vi "Analyze.vi"(8 "error in (no error)":errorcluster, 10 "Image in":T1, 11 "Analyze SecondMomentum in":refnum<class "Analyze SecondMomentum.lvclass">) -> (0 "error out":errorcluster, 1 "Result":refnum<class "Analyze Results Base.lvclass">, 2 "Image out":T1, 3 "Analyze SecondMomentum out":refnum<class "Analyze SecondMomentum.lvclass">)   [LabVIEW 2014, in "Analyze.lvlib" / "Analyze SecondMomentum.lvclass"]
uses:
  Analyze SecondMomentum.lvclass
  <vilib>/vision/Image Controls.llb/IMAQ Image.ctl
  Results and Overlays/Results Base/Analyze Results Base.lvclass
  Results and Overlays/Results Second Momentum/Analyze Results Second Momentum.lvclass
  Results and Overlays/Results Second Momentum/Analyze Results Second Momentum.lvclass/Analyze Results Second Momentum.ctl
  Results and Overlays/Results Second Momentum/Write 1st M x 1.vi
  Results and Overlays/Results Second Momentum/Write 1st M y 1.vi
  Results and Overlays/Results Second Momentum/Write 2nd M x 1.vi
  Results and Overlays/Results Second Momentum/Write 2nd M y 1.vi
  Results and Overlays/Results Second Momentum/Write D x 1.vi
  Analyze BaseClass/Analyze BaseClass/Analyze BaseClass.lvclass
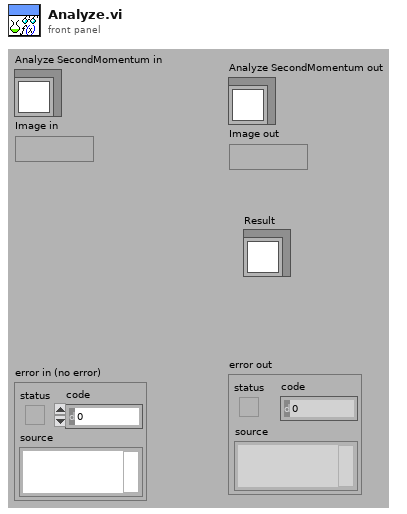
[diagram p1: front panel]
types:
  T1 = typedef "IMAQ Image.ctl" = refnum<image>
  T2 = typedef "ROI Descriptor" = cluster{"Global Rectangle":i32[], "Contours":cluster{"ID":enum32{"External", "Internal"}, "Type":u32, "Coordinates":i32[]}[]}
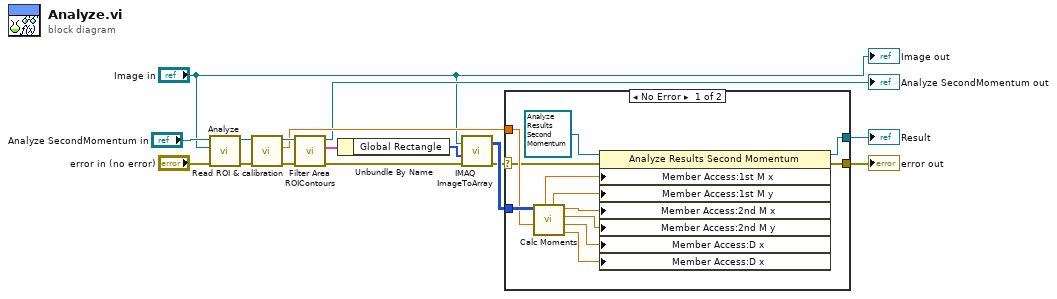
[diagram p0: block diagram]
diagram:
  n1 = call-parent "Analyze.vi"("error in (no error)"="error in (no error)", "Image in"="Image in", "Analyze BaseClass in"="Analyze SecondMomentum in") -> ("error out"=w6:errorcluster, "Analyze BaseClass out"=w5:refnum<class "Analyze SecondMomentum.lvclass">)  [unwired: 5 in, 2 out]
  n2 = call-dynamic "Read ROI & calibration.vi"("error in (no error)"=w6, "Analyze BaseClass in"=w5) -> ("error out"=w16:errorcluster, "calibration mm/px"=w13:dbl[unit], "Analyze BaseClass out"=w15:refnum<class "Analyze SecondMomentum.lvclass">)  [unwired: 6 in, 1 out]
  n3 = call-dynamic "Filter Area ROIContours.vi"("error in (no error)"=w16, "Analyze BaseClass in"=w15) -> ("error out"=w12:errorcluster, "ROI of Area type"=w11:T2, "Analyze BaseClass out"=→"Analyze SecondMomentum out":refnum<class "Analyze SecondMomentum.lvclass">)  [unwired: 7 in]
  n4 = Unbundle By Name(w11) -> ("Global Rectangle"=w10:i32[])
  n5 = call "IMAQ ImageToArray"("error in (no error)"=w12, "Optional Rectangle"=w10, "Image"="Image in") -> ("error out"=w3:errorcluster, "Image Pixels (I16)"=w9:i16[][])  [unwired: 1 in, 3 out]
  n6 = case shown="No Error" w3 {
    selector: w3 -> [w18 w29]
    tunnel: [w17 w29] -> w14
    tunnel: w13 -> [w20 _]
    tunnel: w9 -> [w28 _]
    tunnel: [w19 _] -> w4
    frame No Error {
      n7 = call "Calc Moments.vi"("Calibration"=w20, "image array"=w28) -> ("Durchmesser Y"=w21:dbl[unit], "Durchmesser X"=w22:dbl[unit], "2nd Moment y"=w23:dbl[unit], "2nd Moment x"=w24:dbl[unit], "1st Moment y"=w25:dbl[unit], "1st Moment x"=w26:dbl[unit])  [unwired: 4 in]
      n8 = property class="Analyze Results Second Momentum"(reference=refnum<class "Analyze Results Second Momentum.lvclass"> refnum ("Analyze Results Second Momentum.lvclass"), error in=w18, "Member Access:1st M x"=w26, "Member Access:1st M y"=w25, "Member Access:2nd M x"=w24, "Member Access:2nd M y"=w23, "Member Access:D x"=w22, "Member Access:D x"=w21) -> (reference out=w19:refnum<class "Analyze Results Second Momentum.lvclass">, error out=w17:errorcluster)
    }
    frame Error {
    }
  }
  "error out" <- w14
  "Result" <- w4
  "Image out" <- "Image in"
